vi "Set Stream Speed and Acceleration (FW7).vi"(5 "Centripetal Acceleration (0)":u64, 6 "Maximum Speed (0)":u64, 7 "Tangential Acceleration (0)":u64, 8 "error in (no error)":errorcluster, 9 "Device Number":string, 10 "Stream Number (1)":u8=1, 11 "VISA resource name":refnum<visa-resource-name>) -> (0 "error out":errorcluster, 3 "VISA resource name out":refnum<visa-resource-name>)   [LabVIEW 2013, in "Zaber A Series.lvlib"]
doc: "Change the maximum speed and acceleration parameters of an open stream. This command does not take effect until any other commands already in the stream have been completed.\n\nSpeed and accleration inputs are in device units. Use the Convert Velocity/Acceleration Units to Device Units VIs to convert from standard units of measure. A value of 0 for Maximum Speed, Tangential Acceleration, or Centripetal Acceleration will leave that property unchanged.\n\nThis VI does not check in advance for error conditions such as streams not being supported.\n\nThis VI requires that the Initialize VI has been called with the same serial port."
uses:
  Zaber A Series.lvlib
  Private/All Commands.ctl
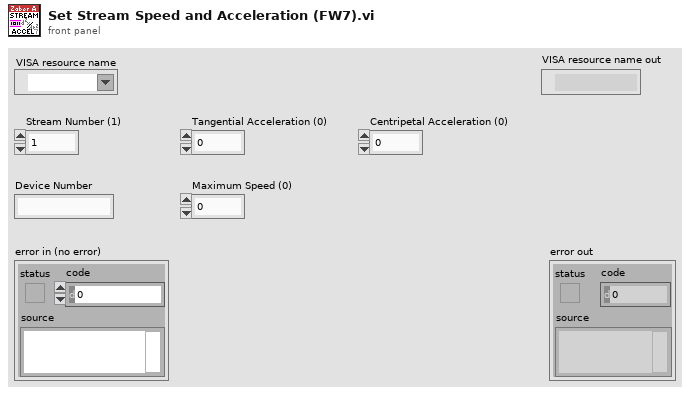
[diagram p1: front panel]
types:
  T1 = typedef "Zaber A Series.lvlib/All Commands.ctl" = string
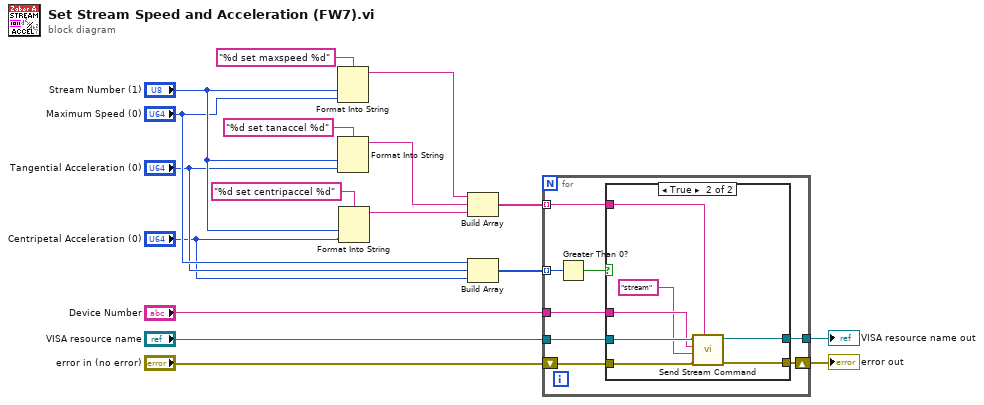
[diagram p0: block diagram]
diagram:
  n1 = Format Into String(format string="%d set maxspeed %d", "Stream Number (1)", "Maximum Speed (0)") -> (resulting string=w10:string)  [unwired: 2 in, 1 out]
  n2 = Format Into String(format string="%d set tanaccel %d", "Stream Number (1)", "Tangential Acceleration (0)") -> (resulting string=w9:string)  [unwired: 2 in, 1 out]
  n3 = Format Into String(format string="%d set centripaccel %d", "Stream Number (1)", "Centripetal Acceleration (0)") -> (resulting string=w8:string)  [unwired: 2 in, 1 out]
  n4 = Build Array(w10, w9, w8) -> (w17:string[])
  n5 = Build Array("Maximum Speed (0)", "Tangential Acceleration (0)", "Centripetal Acceleration (0)") -> (w1:u64[])
  n6 = for {
    tunnel: w17 -> [w23] mode=indexing
    tunnel: "VISA resource name" -> [w25]
    tunnel: [w22] -> w3
    tunnel: "Device Number" -> [w20]
    shift-right: [w21] -> w2
    shift-left: "error in (no error)" -> [w24]
    tunnel: w1 -> [w19] mode=indexing
    n7 = Greater Than 0?(x=w19) -> (x > 0?=w18:bool)
    n8 = case shown="True" w18 {
      tunnel: w25 -> [w27 w34]
      tunnel: w24 -> [w26 w33]
      tunnel: w23 -> [_ w30]
      tunnel: [w27 w32] -> w22
      tunnel: [w26 w31] -> w21
      tunnel: w20 -> [_ w29]
      frame False {
      }
      frame True {
        n9 = call "Send Stream Command.vi"("Data"=w30, "error in (no error)"=w33, "Command"=T1 "stream" ("Complete Command List"), "Device Number"=w29, "VISA resource name"=w34) -> ("error out"=w31:errorcluster, "VISA resource name out"=w32:refnum<visa-resource-name>)  [unwired: 5 in]
      }
    }
  }
  "VISA resource name out" <- w3
  "error out" <- w2
